vi "SlideTiles.vi"(7 "Side":T1=enum."left", 8 "error in (no error)":errorcluster, 10 "Tilecodes":u32[](array[numeric]), 11 "Game in":refnum<class "Game.lvclass">) -> (0 "error out":errorcluster, 3 "Game out":refnum<class "Game.lvclass">)   [LabVIEW 2019, in "RT_Game.lvlib" / "Game.lvclass"]
uses:
  Game.lvclass
  ScreenSide.ctl
  Engine/MessageCluster.ctl
  SlideJob.ctl
  Game.lvclass/Game.ctl
  Engine/Engine.lvclass
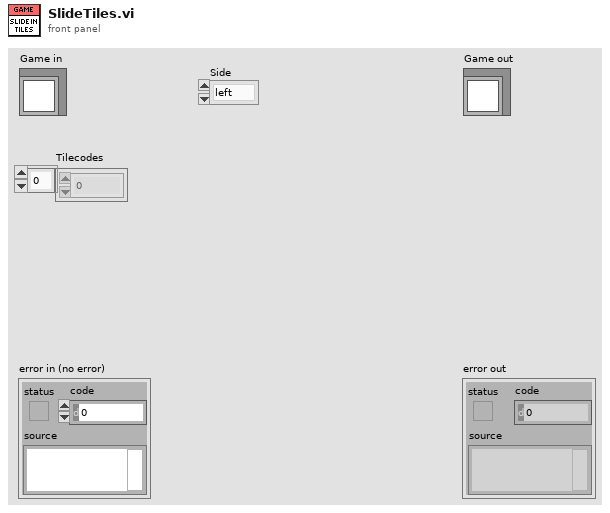
[diagram p1: front panel]
types:
  T1 = typedef "RT_Game.lvlib/Game.lvclass/ScreenSide.ctl" = enum16{"up", "down", "left", "right", "none"}
  T2 = typedef "RT_Game.lvlib/Engine.lvclass/SlideJob.ctl" = cluster{"Pixel":u32[], "Side":T1}
  T3 = typedef "RT_Game.lvlib/Engine.lvclass/MessageCluster.ctl" = cluster{"Message":string, "Data":variant}
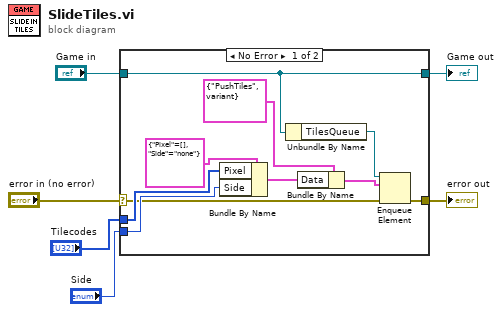
[diagram p0: block diagram]
diagram:
  n1 = case shown="No Error" "error in (no error)" {
    selector: "error in (no error)" -> [w13 w18]
    tunnel: [w12 w18] -> w5
    tunnel: [w14 w17] -> w3
    tunnel: "Game in" -> [w14 w17]
    tunnel: "Side" -> [w16 _]
    tunnel: "Tilecodes" -> [w15 _]
    frame No Error {
      n2 = Bundle By Name(cluster=T2 {"Pixel"=[], "Side"=enum."none"} ("SlideJob"), "Pixel"=w15, "Side"=w16) -> (w7:T2)
      n3 = Unbundle By Name(w14) -> ("TilesQueue"=w11:refnum<queue>)
      n4 = Bundle By Name(cluster=T3 {"Message"="PushTiles", "Data"=variant} ("element"), "Data"=w7) -> (w9:T3)
      n5 = Enqueue Element(queue=w11, element=w9, error in (no error)=w13) -> (error out=w12:errorcluster)  [unwired: 1 in, 2 out]
    }
    frame Error {
    }
  }
  "error out" <- w5
  "Game out" <- w3
